vi "Set Shutter.vi"(7 "openingtime":i32, 8 "error in (no error)":errorcluster, 9 "closingtime":i32, 10 "mode":i32, 11 "typ":i32) -> (0 "error out":errorcluster, 3 "function return":u32)   [LabVIEW 2014, in "atmcd32d.lvlib"]
doc: "unsigned int WINAPI SetShutter(int typ, int mode, int closingtime, int openingtime);"
uses:
  atmcd32d.lvlib
  atmcd32d.dll
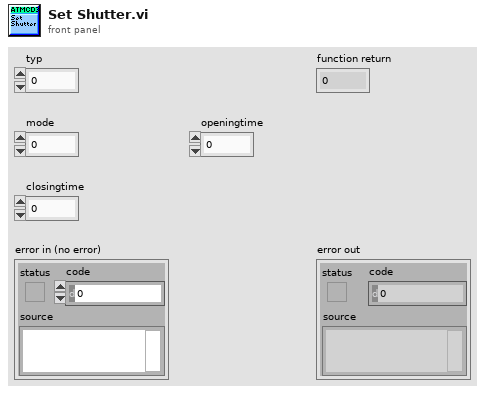
[diagram p1: front panel]
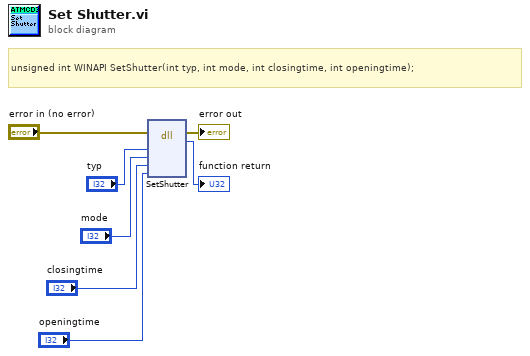
[diagram p0: block diagram]
diagram:
  # "unsigned int WINAPI SetShutter(int typ, int mode, int closingtime, int openingtime);"
  n1 = dll-call lib="C:/Users/Bakir/Documents/Lambda2-Testing/lib/Andorlib/atmcd32d.*" fn="SetShutter"(error in="error in (no error)", "typ"="typ", "mode"="mode", "closingtime"="closingtime", "openingtime"="openingtime") -> (error out=→"error out":errorcluster, →"function return":u32)  [unwired: 6 in, 1 out]
